vi "Control Digital Output - PWM - Initialize.vi"(0 "frequency":dbl=1.0 format="%.6f", 5 "duty cycle":dbl=0.5 format="%.6f", 7 "counter input":tag, 9 "DAQmx Terminal":tag, 11 "Error In":errorcluster) -> (4 "task out":refnum<k21>, 15 "Error Out":errorcluster)   [LabVIEW 2016]
uses:
  <vilib>/DAQmx/create/channels.llb/DAQmx Create Channel (CO-Pulse Generation-Frequency).vi
  <vilib>/DAQmx/configure/timing.llb/DAQmx Timing (Implicit).vi
  <resource>/objmgr/daqmx.rc
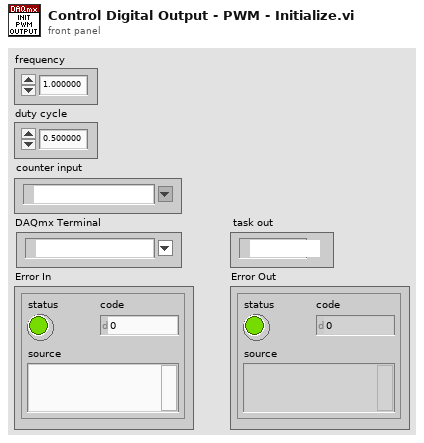
[diagram p1: front panel]
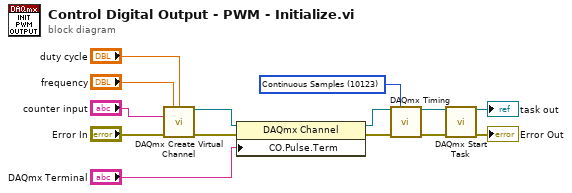
[diagram p0: block diagram]
diagram:
  w13 = 10123 items=["Finite Samples"=10178, "Continuous Samples"=10123, "Hardware Timed Single Point"=12522] ("sample mode")
  n1 = call-poly <vilib>:"DAQmx Create Virtual Channel.vi"("frequency"="frequency", "duty cycle"="duty cycle", "counter"="counter input", "error in"="Error In") -> ("task out"=w14:refnum<k21>, "error out"=w10:errorcluster)  [unwired: 10 in]
  n2 = property class="DAQmx Channel"(reference=w14, error in=w10, "CO.Pulse.Term"="DAQmx Terminal") -> (reference out=w12:refnum<k21>, error out=w11:errorcluster)
  n3 = call-poly <vilib>:"DAQmx Timing.vi"("task/channels in"=w12, "sample mode"=w13, "error in"=w11) -> ("task out"=w5:refnum<k21>, "error out"=w2:errorcluster)  [unwired: 11 in]
  n4 = call <vilib>:"DAQmx Start Task.vi"("task/channels in"=w5, "error in"=w2) -> ("task out"=→"task out":refnum<k21>, "error out"=→"Error Out":errorcluster)  [unwired: 12 in]
